vi "Pac Man (top vi.).vi"() -> ()   [LabVIEW 2014]
uses:
  <vilib>/Utility/inputDevices.llb/keyboardAcquire.vi
  <vilib>/Utility/inputDevices.llb/closeKeyboard.vi
panel:
  in  "W/L":i32
  out "Player\nname":string
  out "Time":string
  in  "stop 3":bool
  out "Points":i32
  out "?":u32[][](array[colorbox])
  in  "stop":bool
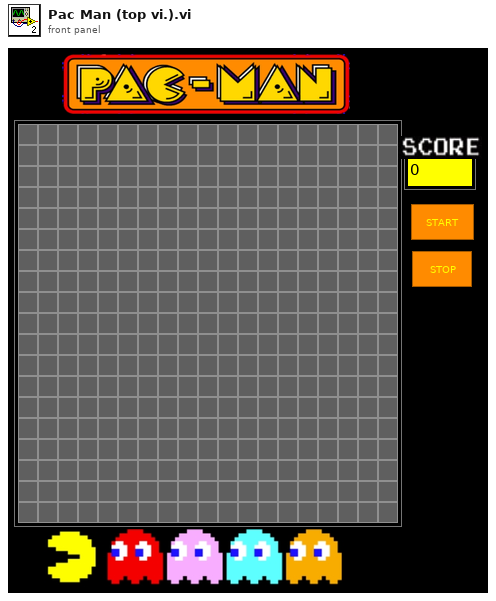
[diagram p1: front panel]
types:
  T1 = enum16{"0", "1", "2", "3", "4", "5", "6", "7", "8", "9", "A", "B", "C", "D", "E", "F", "G", "H", "I", "J", "K", "L", "M", "N", "O", "P", "Q", "R", "S", "T", "U", "V", "W", "X", "Y", "Z", "F1", "F2", "F3", "F4", "F5", "F6", "F7", "F8", "F9", "F10", "F11", "F12", "F13", "F14", "F15", "ADD", "BACK", "BACKSLASH", "CAPITAL", "COMMA", "DECIMAL", "DELETE", "DIVIDE", "DOWN", "END", "EQUALS", "ESCAPE", "GRAVE (`)", "HOME", "INSERT", "LBRACKET", "LCONTROL", "LEFT", "L ALT", "LSHIFT", "LWIN", "MINUS", "MULTIPLY", "NEXT", "NUMLOCK", "NUMPAD_0", "NUMPAD_1", "NUMPAD_2", "NUMPAD_3", "NUMPAD_4", "NUMPAD_5", "NUMPAD_6", "NUMPAD_7", "NUMPAD_8", "NUMPAD_9", "PAUSE", "PERIOD", "PRIOR (PG UP)", "RBRACKET", "RCONTROL", "RETURN", "RIGHT", "R ALT", "RSHIFT", "RWIN", "SCROLL", "SEMICOLON", "SLASH", "SPACE", "SUBTRACT", "TAB", "UP", "ENTER (num pad)", "' (quote)"}[]
  T2 = enum16{"0", "1", "2", "3", "4", "5", "6", "7", "8", "9", "A", "B", "C", "D", "E", "F", "G", "H", "I", "J", "K", "L", "M", "N", "O", "P", "Q", "R", "S", "T", "U", "V", "W", "X", "Y", "Z", "F1", "F2", "F3", "F4", "F5", "F6", "F7", "F8", "F9", "F10", "F11", "F12", "F13", "F14", "F15", "ADD", "BACK", "BACKSLASH", "CAPITAL", "COMMA", "DECIMAL", "DELETE", "DIVIDE", "DOWN", "END", "EQUALS", "ESCAPE", "GRAVE (`)", "HOME", "INSERT", "LBRACKET", "LCONTROL", "LEFT", "L ALT", "LSHIFT", "LWIN", "MINUS", "MULTIPLY", "NEXT", "NUMLOCK", "NUMPAD_0", "NUMPAD_1", "NUMPAD_2", "NUMPAD_3", "NUMPAD_4", "NUMPAD_5", "NUMPAD_6", "NUMPAD_7", "NUMPAD_8", "NUMPAD_9", "PAUSE", "PERIOD", "PRIOR (PG UP)", "RBRACKET", "RCONTROL", "RETURN", "RIGHT", "R ALT", "RSHIFT", "RWIN", "SCROLL", "SEMICOLON", "SLASH", "SPACE", "SUBTRACT", "TAB", "UP", "ENTER (num pad)", "' (quote)"}
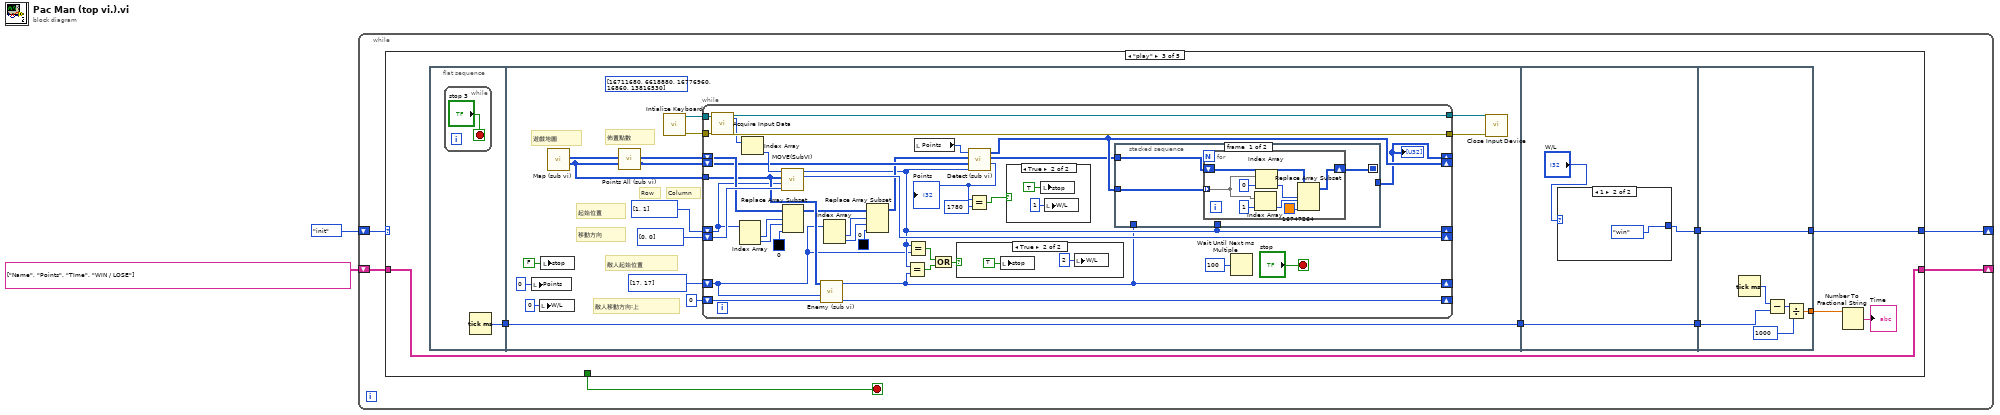
[diagram p0: block diagram]
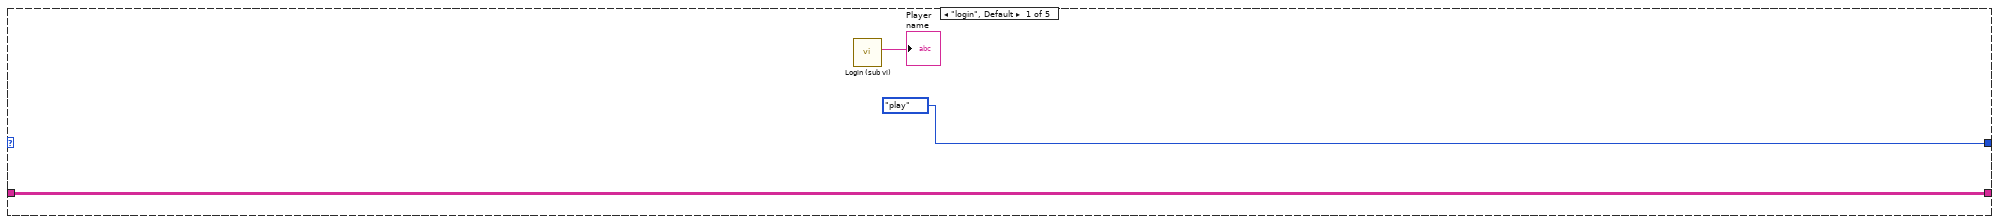
[diagram p2: hidden frame]
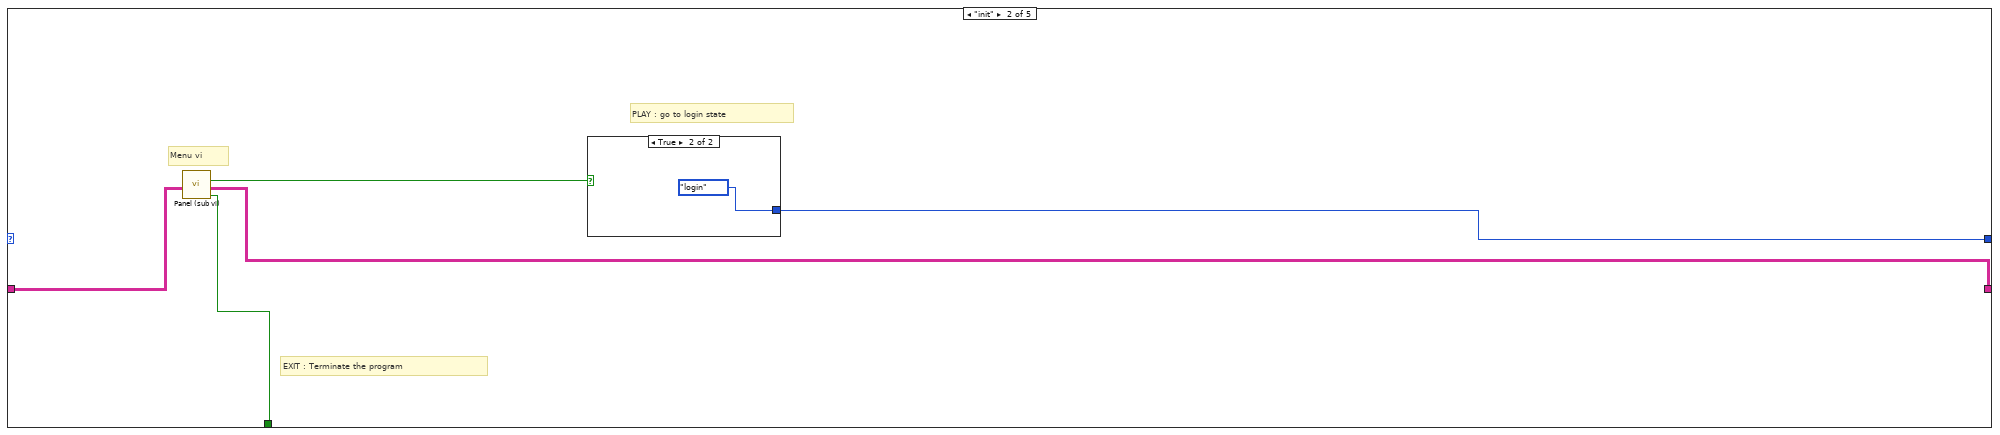
[diagram p3: hidden frame]
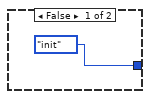
[diagram p4: hidden frame]
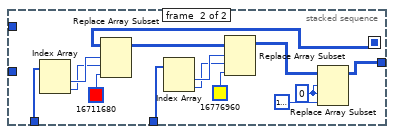
[diagram p7: hidden frame]
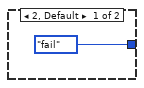
[diagram p8: hidden frame]
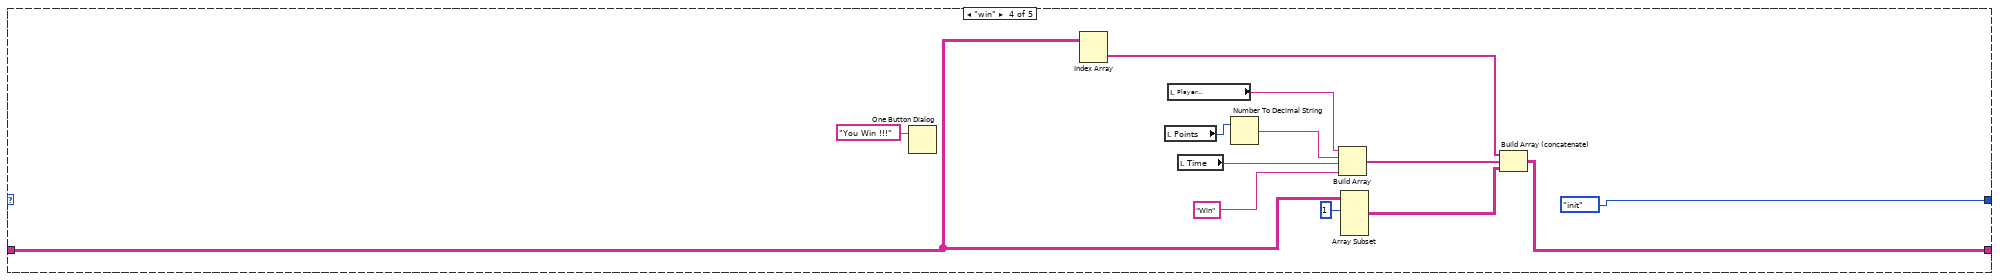
[diagram p9: hidden frame]
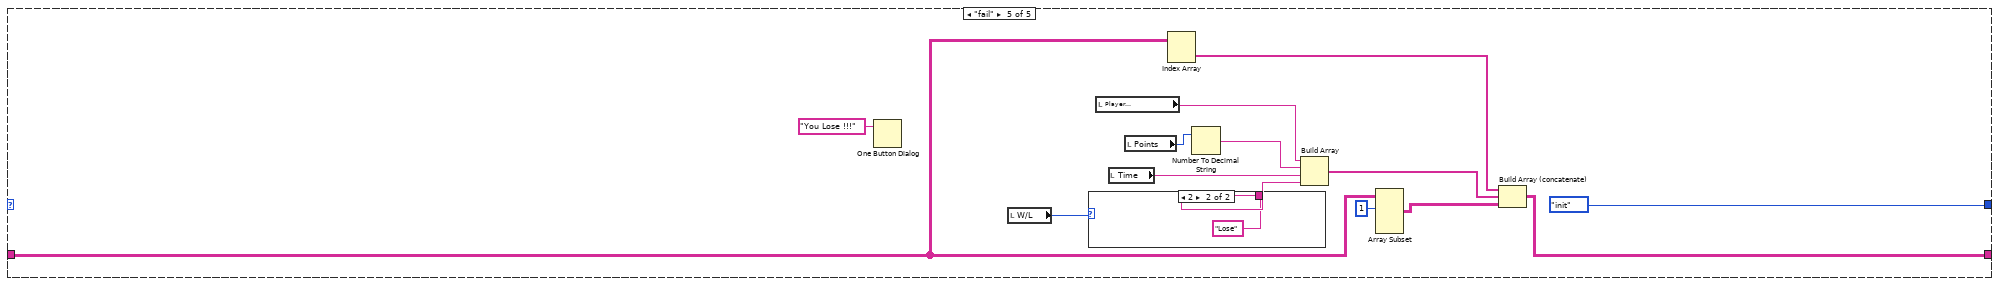
[diagram p10: hidden frame]
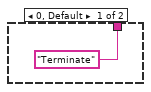
[diagram p11: hidden frame]
diagram:
  n1 = while {
    shift-right: [w6] -> _
    shift-left: enum16{"login", "init", "play", "win", "fail"}."init" -> [w7]
    shift-right: [w4] -> _
    shift-left: string[][] [["Name", "Points", "TIme", "WIN / LOSE"]] -> [w5]
    stop <- w3 stop-if-true
    n2 = case shown="\"play\"" w7 {
      tunnel: [enum16{"login", "init", "play", "win", "fail"}."play" w15 w25 enum16{"login", "init", "play", "win", "fail"}."init" enum16{"login", "init", "play", "win", "fail"}."init"] -> w6
      tunnel: w5 -> [w8 w12 w21 w126 w139]
      tunnel: [w8 w13 w21 w128 w142] -> w4
      tunnel: [_ w11 _ _ _] -> w3
      frame "login", Default {
        n3 = call "Login (sub vi).vi"() -> ("Player\nname 2"=→"Player\nname":string)  [unwired: 11 in]
      }
      frame "init" {
        # "PLAY : go to login state"
        # "EXIT : Terminate the program"
        # "Menu vi"
        n4 = call "Panel (sub vi).vi"("Record"=w12) -> ("EXIT 2"=w11:bool, "Record"=w13:string[][], "PLAY 2"=w14:bool)  [unwired: 8 in]
        n5 = case shown="True" w14 {
          tunnel: [enum16{"login", "init", "play", "win", "fail"}."init" enum16{"login", "init", "play", "win", "fail"}."login"] -> w15
          frame False {
          }
          frame True {
          }
        }
      }
      frame "play" {
        n6 = flat-sequence {
          tunnel: [w26] -> w24
          tunnel: [w33] -> w19
          tunnel: w24 -> [w33]
          tunnel: [w110] -> w20
          tunnel: w19 -> [w112]
          tunnel: [w112] -> w18
          tunnel: [w120] -> w25
          tunnel: w20 -> [w120]
          tunnel: w18 -> [w118]
          tunnel: [w115] -> w23
          frame #0 {
            n7 = while {
              stop <- "stop 3" stop-if-true
            }
            n8 = Tick Count (ms)() -> (millisecond timer value=w26:u32)
          }
          frame #1 {
            (unwired) u32[] [16711680, 6618880, 16776960, 16860, 13816530]
            # "敵人移動方向:上"
            # "敵人起始位置"
            # "佈置點數"
            # "移動方向"
            # "起始位置"
            # "遊戲地圖"
            # "Column"
            # "Row"
            n9 = local write "Points"(0 ("Points")) -> ()
            n10 = local write "W/L"(0 ("W/L")) -> ()
            n11 = local write "stop"(FALSE ("stop")) -> ()
            n12 = call "Map (sub vi).vi"() -> ("Position"=w30:i32[][], "Display"=w31:u32[][])  [unwired: 10 in]
            n13 = call "Points All (sub vi).vi"("Boarder"=w30, "Display"=w31) -> ("Points position"=w28:i32[][], "Display 2"=w29:u32[][])  [unwired: 8 in]
            n14 = call <vilib>:"Intialize Keyboard.vi"() -> ("error out"=w42:errorcluster, "device ID"=w43:refnum<k1>)  [unwired: 10 in]
            n15 = while {
              tunnel: w43 -> [w80]
              tunnel: w42 -> [w79]
              tunnel: [w78] -> w41
              tunnel: [w77] -> w36
              shift-right: [w52] -> _
              shift-left: i32[] [1, 1] -> [w50]
              shift-right: [w74] -> _
              shift-left: i32[] [0, 0] -> [w71]
              tunnel: w30 -> [w65]
              shift-right: [w54] -> _
              shift-left: w29 -> [w67]
              shift-right: [w56] -> _
              shift-left: w28 -> [w62]
              shift-right: [w51] -> _
              shift-left: i32[] [17, 17] -> [w49]
              shift-right: [w63] -> _
              shift-left: 0 -> [w64]
              stop <- "stop" stop-if-true
              n16 = call-poly <vilib>:"Acquire Input Data.vi"("device ID"=w80, "error in (no error)"=w79) -> ("device ID"=w77:refnum<k1>, "keys pressed"=w76:T1, "error out"=w78:errorcluster)  [unwired: 15 in]
              n17 = Index Array(array=w50) -> (element #1=w69:i32, element #2=w68:i32)  [unwired: 2 in]
              n18 = Index Array(array=w76) -> (element=w75:T2)  [unwired: 1 in]
              n19 = call "MOVE(SubVI).vi"("Move Direction"=w71, "former position"=w50, "boarder"=w65, "key in"=w75) -> ("Move Direction out"=w74:i32[], "position"=w52:i32[])  [unwired: 6 in]
              n20 = Replace Array Subset(array=w67, new element=u32 0 ("Color Box"), index (row)=w69, index (col)=w68) -> (w58:u32[][])
              n21 = call "Enemy (sub vi).vi"("Direct in"=w64, "position in"=w49, "boarder"=w65) -> ("Direct out"=w63:i32, "position out"=w51:i32[])  [unwired: 7 in]
              n22 = Index Array(array=w49) -> (element #1=w60:i32, element #2=w59:i32)  [unwired: 2 in]
              n23 = Replace Array Subset(array=w58, new element=u32 0 ("Color Box"), index (row)=w60, index (col)=w59) -> (w57:u32[][])
              n24 = Equal?(x=w52, y=w51) -> (x = y?=w47:bool)
              n25 = Equal?(x=w52, y=w49) -> (x = y?=w48:bool)
              n26 = local read "Points"() -> (w66:i32)
              n27 = Compound Arithmetic op=OR(w48, w47) -> (w53:bool)
              n28 = case shown="True" w53 {
                frame False {
                }
                frame True {
                  n29 = local write "stop"(TRUE ("stop")) -> ()
                  n30 = local write "W/L"(2 ("W/L")) -> ()
                }
              }
              n31 = call "Detect (sub vi).vi"("MOVE position"=w52, "Points position"=w62, "Display"=w57, "Points"=w66) -> ("Points 2"=w44:i32, "Display 2"=w55:u32[][], "Points position 2"=w56:i32[][])  [unwired: 5 in]
              "Points" <- w44
              n32 = Equal?(x=w44, y=1780) -> (x = y?=w46:bool)
              n33 = case shown="True" w46 {
                frame False {
                }
                frame True {
                  n34 = local write "stop"(TRUE ("stop")) -> ()
                  n35 = local write "W/L"(1 ("W/L")) -> ()
                }
              }
              n36 = stacked-sequence {
                seq-local: [w85 _] -> [_ w107]
                tunnel: w56 -> [w87 _]
                tunnel: w55 -> [w86 _]
                tunnel: [_ w98] -> w54
                tunnel: w51 -> [_ w105]
                tunnel: w52 -> [_ w102]
                frame #0 {
                  n37 = for {
                    shift-right: [w91] -> w85
                    shift-left: w86 -> [w92]
                    tunnel: w87 -> [w90] mode=indexing
                    n38 = Index Array(array=w90, index=1) -> (element=w88:i32)
                    n39 = Index Array(array=w90, index=0) -> (element=w89:i32)
                    n40 = Replace Array Subset(array=w92, new element=u32 16747264 ("Color Box"), index (row)=w89, index (col)=w88) -> (w91:u32[][])
                  }
                }
                frame #1 {
                  w97 = 0 ("disabled index (col)")
                  n41 = Index Array(array=w105) -> (element #1=w104:i32, element #2=w103:i32)  [unwired: 2 in]
                  n42 = Replace Array Subset(array=w107, new element=u32 16711680 ("Color Box"), index (row)=w104, index (col)=w103) -> (w106:u32[][])
                  n43 = Index Array(array=w102) -> (element #1=w101:i32, element #2=w100:i32)  [unwired: 2 in]
                  n44 = Replace Array Subset(array=w106, new element=u32 16776960 ("Color Box"), index (row)=w101, index (col)=w100) -> (w99:u32[][])
                  n45 = Replace Array Subset(array=w99, new element=u32 16777224 ("Color Box"), index (row)=w97, index (col)=w97) -> (w98:u32[][])
                }
              }
              "?" <- w54
              n46 = Wait Until Next ms Multiple(millisecond multiple=u32 100) -> ()  [unwired: 1 out]
            }
            n47 = call-poly <vilib>:"Close Input Device.vi"("error in (no error)"=w41, "device ID"=w36) -> ()  [unwired: 8 in, 1 out]
          }
          frame #2 {
            n48 = case shown="1" "W/L" {
              tunnel: [enum16{"login", "init", "play", "win", "fail"}."fail" enum16{"login", "init", "play", "win", "fail"}."win"] -> w110
              frame 2, Default {
              }
              frame 1 {
              }
            }
          }
          frame #3 {
            n49 = Tick Count (ms)() -> (millisecond timer value=w119:u32)
            n50 = Subtract(x=w119, y=w118) -> (x-y=w117:u32)
            n51 = Divide(x=w117, y=u32 1000) -> (x/y=w115:dbl)
          }
        }
        n52 = Number To Fractional String(number=w23) -> (F-format string=→"Time":string)  [unwired: 3 in]
      }
      frame "win" {
        n53 = One Button Dialog(message="You Win !!!") -> ()  [unwired: 1 in, 1 out]
        n54 = Index Array(array=w126) -> (element=w123:string[])  [unwired: 2 in]
        n55 = local read "Points"() -> (w127:i32)
        n56 = local read "Player\nname"() -> (w129:string)
        n57 = local read "Time"() -> (w131:string)
        n58 = Number To Decimal String(number=w127) -> (decimal integer string=w130:string)  [unwired: 1 in]
        n59 = Build Array(w129, w130, w131, "Win" ("element")) -> (w132:string[])
        n60 = Array Subset(array=w126, index (row)=1 ("index")) -> (w124:string[][])  [unwired: 3 in]
        n61 = Build Array (concatenate)(w123, w132, w124) -> (w128:string[][])
      }
      frame "fail" {
        n62 = One Button Dialog(message="You Lose !!!") -> ()  [unwired: 1 in, 1 out]
        n63 = local read "W/L"() -> (w134:i32)
        n64 = case shown="2" w134 {
          tunnel: ["Terminate" ("element") "Lose" ("element")] -> w140
          frame 0, Default {
          }
          frame 2 {
          }
        }
        n65 = local read "Player\nname"() -> (w145:string)
        n66 = local read "Time"() -> (w144:string)
        n67 = local read "Points"() -> (w141:i32)
        n68 = Index Array(array=w139) -> (element=w138:string[])  [unwired: 2 in]
        n69 = Number To Decimal String(number=w141) -> (decimal integer string=w146:string)  [unwired: 1 in]
        n70 = Build Array(w145, w146, w144, w140) -> (w143:string[])
        n71 = Array Subset(array=w139, index (row)=1 ("index")) -> (w136:string[][])  [unwired: 3 in]
        n72 = Build Array (concatenate)(w138, w143, w136) -> (w142:string[][])
      }
    }
  }
